vi "awgn_channel.vi"(4 "error in (no error)":errorcluster, 6 "noise power (dB)":dbl, 7 "input":cdb[](array[numeric])) -> (0 "error out":errorcluster, 3 "output":cdb[](array[numeric]))   [LabVIEW 2013]
uses:
  <vilib>/Analysis/NI_AALBase.lvlib
panel:
  # "Applies AWGN Channel to input"
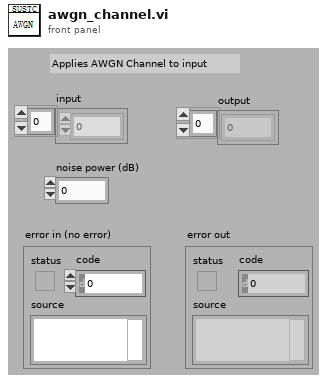
[diagram p1: front panel]
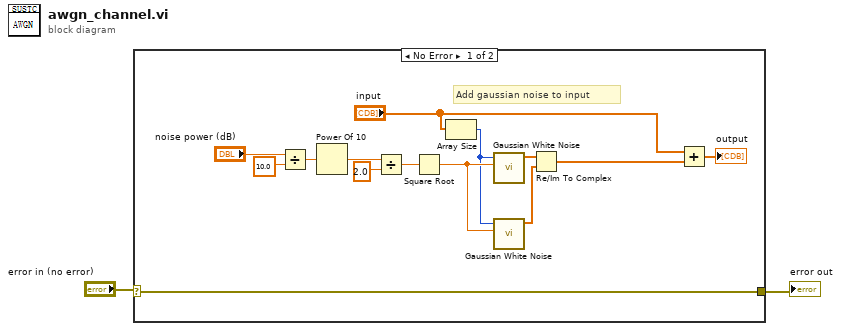
[diagram p0: block diagram]
diagram:
  n1 = case shown="No Error" "error in (no error)" {
    selector: "error in (no error)" -> [w3 w17]
    tunnel: [w3 w17] -> w1
    frame No Error {
      # "Add gaussian noise to input"
      n2 = Divide(x="noise power (dB)", y=10.0) -> (x/y=w16:dbl)
      n3 = Power Of 10(x=w16) -> (10^x=w11:dbl)
      n4 = Divide(x=w11, y=2.0) -> (x/y=w12:dbl)
      n5 = Square Root(x=w12) -> (sqrt(x)=w10:dbl)
      n6 = Array Size(array="input") -> (size(s)=w9:i32)
      n7 = call <vilib>:"Gaussian White Noise.vi"("standard deviation"=w10, "samples"=w9) -> ("Gaussian noise pattern"=w6:dbl[])  [unwired: 8 in, 1 out]
      n8 = call <vilib>:"Gaussian White Noise.vi"("standard deviation"=w10, "samples"=w9) -> ("Gaussian noise pattern"=w7:dbl[])  [unwired: 8 in, 1 out]
      n9 = Re/Im To Complex(1:w7, 2:w6) -> (0:w8:cdb[])
      n10 = Add(x="input", y=w8) -> (x+y=→"output":cdb[])
    }
    frame Error {
    }
  }
  "error out" <- w1
